vi "show2dViewer.vi"(6 "nos":u32, 8 "error in (no error)":errorcluster, 9 "camera":u16, 10 "block":u32, 11 "drvno":u32) -> (0 "error out":errorcluster)   [LabVIEW 2015, in "ESLSCDLL.lvlib"]
uses:
  ESLSCDLL.lvlib
  Globals.vi
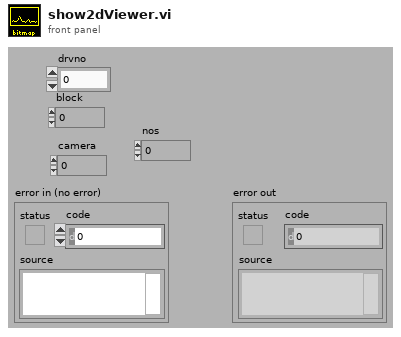
[diagram p1: front panel]
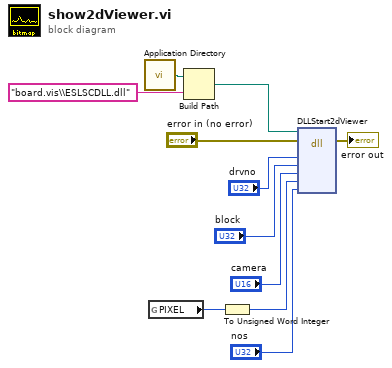
[diagram p0: block diagram]
diagram:
  n1 = call <vilib>:"Application Directory.vi"() -> ("Application Directory"=w5:path)
  n2 = global read "Globals.vi" "PIXEL"() -> (w6:u32)
  n3 = Build Path(base path=w5, name or relative path="board.vis\\ESLSCDLL.dll") -> (appended path=w3:path)
  n4 = To Unsigned Word Integer(number=w6) -> (unsigned 16bit integer=w1:u16)
  n5 = dll-call lib="C:/ENTW/PCIE/LV64/board.vis/ESLSCDLL.dll" fn="DLLStart2dViewer" ("lwlscdll.dll:DLLWriteLongS0")(path in=w3, error in="error in (no error)", "drvno"="drvno", "block"="block", "camera"="camera", "pixel"=w1, "nos"="nos") -> (error out=→"error out":errorcluster)  [unwired: 7 in, 1 out]
